vi "TextFit_Build Size and Sort Char Cluster Array.vi"(8 "Error":errorcluster, 9 "Size To Fit":i32=30, 11 "String":string) -> (0 "Error Out":errorcluster, 1 "Final Size Out":i32=30, 2 "Fit Result Out":T4, 3 "Build Array Out":T1[](array[typedef]))   [LabVIEW 2014]
doc: "Builds Sizes and Sorts the Character Cluster array"
uses:
  Controls/Enum/ENUM RB_Fit Result.ctl
  Controls/Cluster/Cluster_Character Size and Priority Data.ctl
  Controls/String_Picture/String Char Normal.ctl
  Controls/Enum/ENUM_Font Size Select.ctl
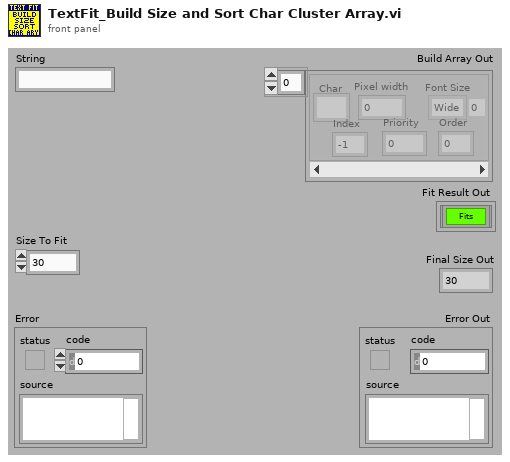
[diagram p1: front panel]
types:
  T1 = typedef "Cluster_Character Size and Priority Data.ctl" = cluster{"Char":T2, "Font Size":T3, "Pixel width":i32, "Priority":i32, "Order":i32, "Index":i32}
  T2 = typedef "String Char Normal.ctl" = string
  T3 = typedef "ENUM_Font Size Select.ctl" = enum16{"Wide", "Med", "Thin"}
  T4 = typedef "ENUM RB_Fit Result.ctl" = enum32{"Fits", "Almost Fits", "NO Fit"}
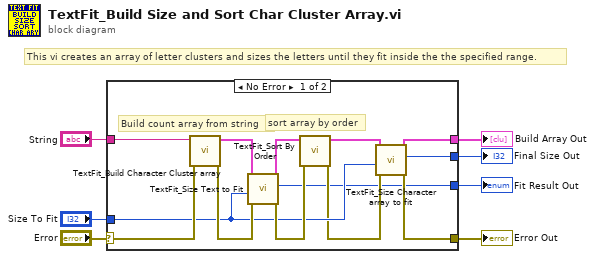
[diagram p0: block diagram]
diagram:
  # "This vi creates an array of letter clusters and sizes the letters until they fit inside the the specified range."
  n1 = case shown="No Error" "Error" {
    selector: "Error" -> [w15 w21]
    tunnel: "String" -> [w20 _]
    tunnel: [w13 _] -> w6
    tunnel: [w10 w21] -> w5
    tunnel: "Size To Fit" -> [w12 _]
    tunnel: [w9 _] -> w2
    tunnel: [w8 _] -> w1
    frame No Error {
      # "sort array by order"
      # "Build count array from string"
      n2 = call "TextFit_Build Character Cluster array.vi"("Error"=w15, "String"=w20) -> ("Error Out"=w19:errorcluster, "Character Array Out"=w17:T1[])  [unwired: 8 in]
      n3 = call "TextFit_Size Text to Fit.vi"("Error"=w19, "Size To Fit"=w12, "Character Array"=w17) -> ("Error Out"=w18:errorcluster, "Fit Result Out"=w9:T4, "Character Array Out"=w16:T1[])  [unwired: 6 in]
      n4 = call "TextFit_Sort By Order.vi"("Error"=w18, "Character Array"=w16) -> ("Error Out"=w11:errorcluster, "Character Array Out"=w14:T1[])  [unwired: 8 in]
      n5 = call "TextFit_Size Character array to fit.vi"("Error"=w11, "Size To Fit"=w12, "Character Array"=w14) -> ("Error Out"=w10:errorcluster, "Pixel Width Out"=w8:i32, "Character Array Out"=w13:T1[])  [unwired: 6 in]
    }
    frame Error {
    }
  }
  "Fit Result Out" <- w2
  "Final Size Out" <- w1
  "Build Array Out" <- w6
  "Error Out" <- w5
